vi "定点周期设置.vi"(4 "每月启动":T1, 6 "每周启动":T2, 7 "Display State In":T3, 8 "测量参数字符串[]":string[](array[string]), 9 "间隔启动":T9, 10 "定点周期":T6, 11 "周期模式":T5) -> (2 "保存输出":bool, 3 "周期设置输出":T8)   [LabVIEW 2016, in "定时设置.xctl"]
uses:
  <vilib>/Utility/miscctls.llb/LVPointTypeDef.ctl
panel:
  out "测试状态.结束时间":timestamp caption="结束时间" format="%<%y/%m/%d %H:%M:%S>T"
  out "测试状态.启动次数":dbl caption="启动次数"
  out "测试状态.启动时间":timestamp caption="启动时间" format="%<%y/%m/%d %H:%M:%S>T"
  in  "测量参数":T4 items=["氨氮"]
  in  "保存":bool
  in  "退出":bool
  in  "批量设置":bool
  out "周期模式选择卡":enum32{"选项卡 1", "选项卡 2"}(tab)
  # "分钟"
  # "次"
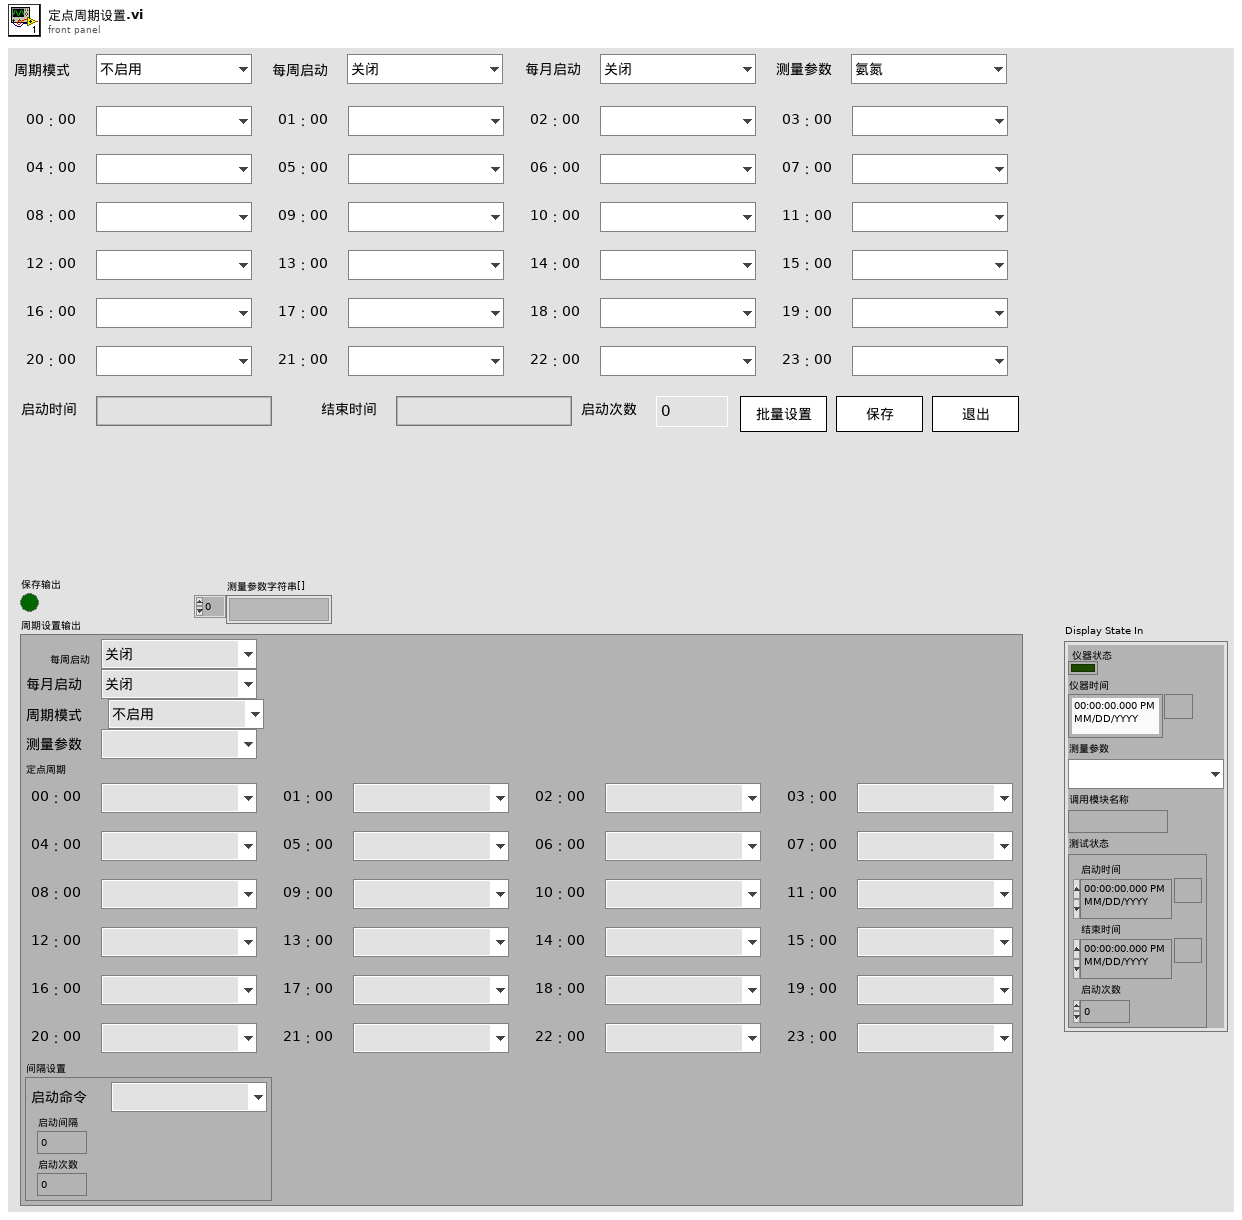
[diagram p1: front panel]
types:
  T1 = typedef "定时设置.xctl/每月启动.ctl" = enum16{"关闭", "1号", "2号", "3号", "4号", "5号", "6号", "7号", "8号", "9号", "10号", "11号", "12号", "13号", "14号", "15号", "16号", "17号", "18号", "19号", "20号", "21号", "22号", "23号", "24号", "25号", "26号", "27号", "28号", "29号", "30号", "31号"}
  T2 = typedef "定时设置.xctl/每周启动.ctl" = enum16{"关闭", "周日", "周一", "周二", "周三", "周四", "周五", "周六"}
  T3 = typedef "定时设置.xctl/状态 1.ctl" = cluster{"仪器状态":bool, "仪器时间":timestamp, "测量参数":T4, "调用模块名称":string, "测试状态":cluster{"启动时间":timestamp, "结束时间":timestamp, "启动次数":dbl}}
  T4 = typedef "定时设置.xctl/测量参数.ctl" = u16
  T5 = typedef "定时设置.xctl/周期模式设置.ctl" = enum16{"不启用", "定点模式", "间隔模式"}
  T6 = typedef "定时设置.xctl/定点周期设置.ctl" = cluster{"启动命令":T7, "启动命令 2":T7, "启动命令 3":T7, "启动命令 4":T7, "启动命令 5":T7, "启动命令 6":T7, "启动命令 7":T7, "启动命令 8":T7, "启动命令 9":T7, "启动命令 10":T7, "启动命令 11":T7, "启动命令 12":T7, "启动命令 13":T7, "启动命令 14":T7, "启动命令 15":T7, "启动命令 16":T7, "启动命令 17":T7, "启动命令 18":T7, "启动命令 19":T7, "启动命令 20":T7, "启动命令 21":T7, "启动命令 22":T7, "启动命令 23":T7, "启动命令 24":T7}
  T7 = typedef "定时设置.xctl/启动命令选择.ctl" = enum16{"", "水样测试", "标样核查", "零点核查", "跨度核查", "空白测试", "平行样测试", "加标回收", "空白校准", "标样校准", "初始化(清洗)"}
  T8 = cluster{"每周启动":T2, "每月启动":T1, "周期模式":T5, "测量参数":T4, "定点周期":T6, "间隔设置":cluster{"启动命令":T7, "启动间隔":dbl, "启动次数":i32}}
  T9 = typedef "定时设置.xctl/间隔启动设置.ctl" = cluster{"启动命令":T7, "启动间隔":dbl, "启动次数":i32}
  T10 = typedef "LVPointTypeDef.ctl" = cluster{"Horizontal":i16, "Vertical":i16}
  T11 = typedef "周期设置.lvlib/周期模式设置.ctl" = enum16{"不启用", "定点模式", "间隔模式"}
  T12 = cluster{"每周启动":T2, "每月启动":T1, "周期模式":T5, "测量参数":T4, "定点周期":T6, cluster{"启动命令":T7, "启动间隔":dbl, "启动次数":i32}}
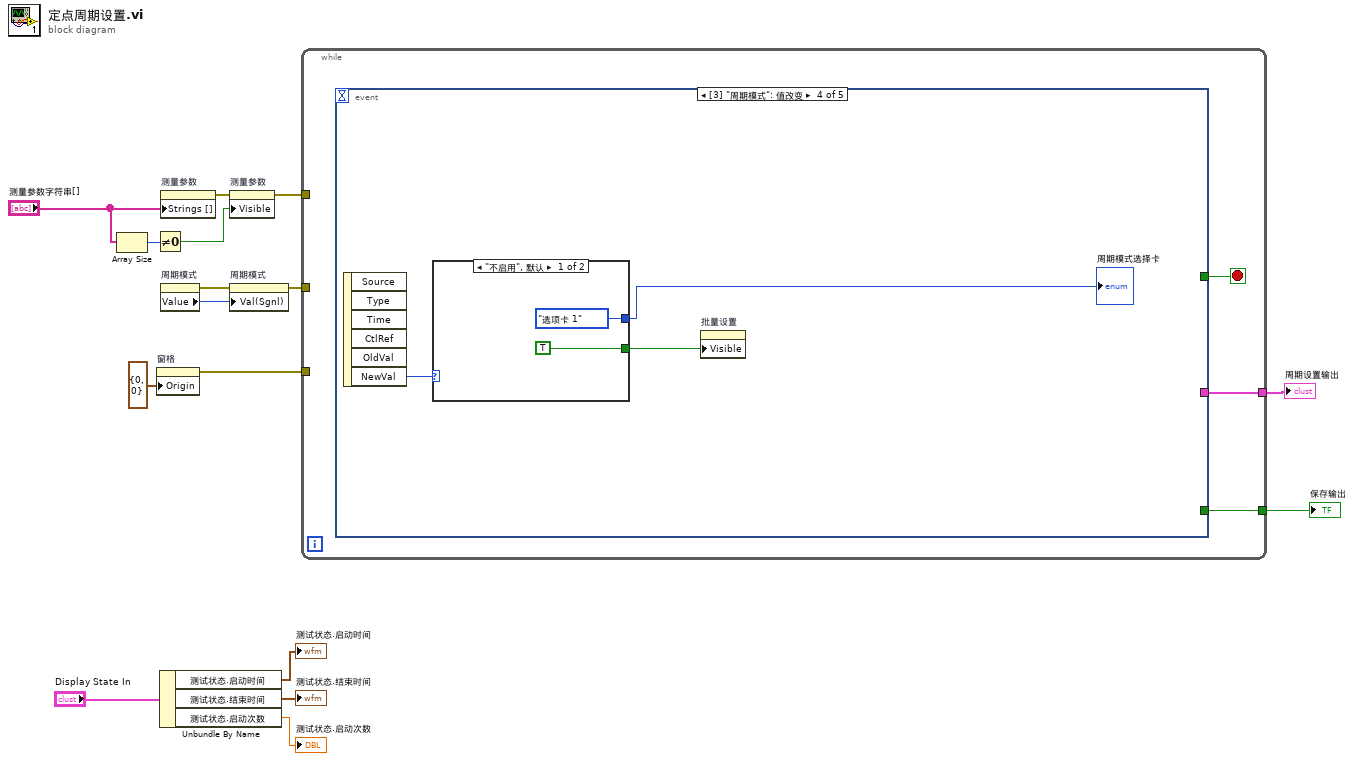
[diagram p0: block diagram]
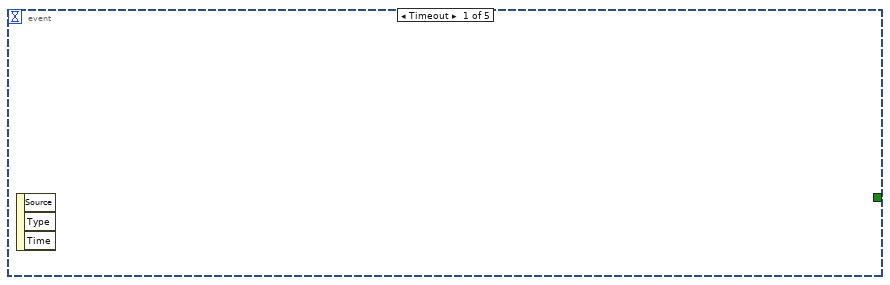
[diagram p2: hidden frame]
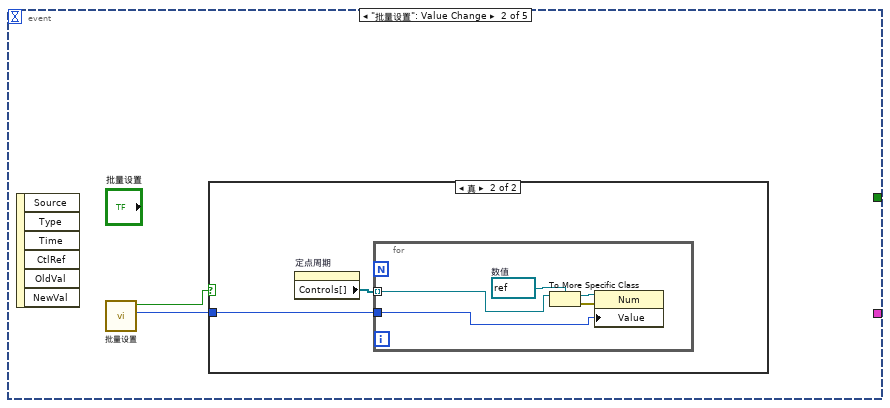
[diagram p3: hidden frame]
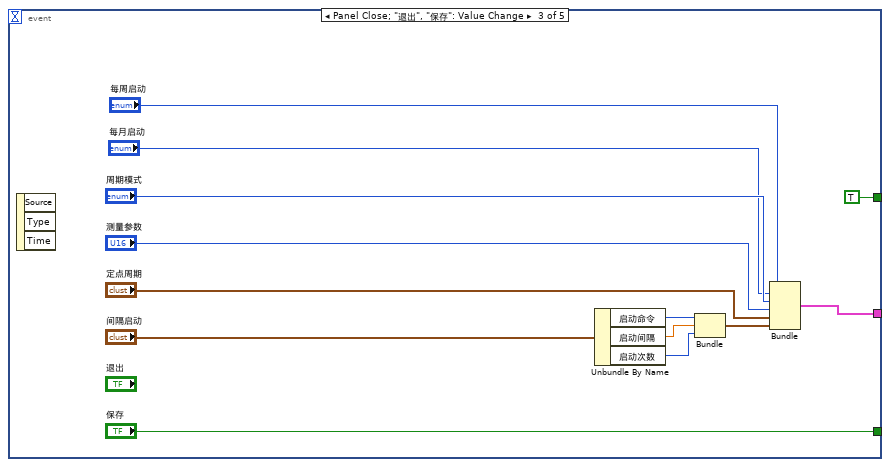
[diagram p5: hidden frame]
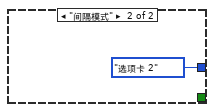
[diagram p6: hidden frame]
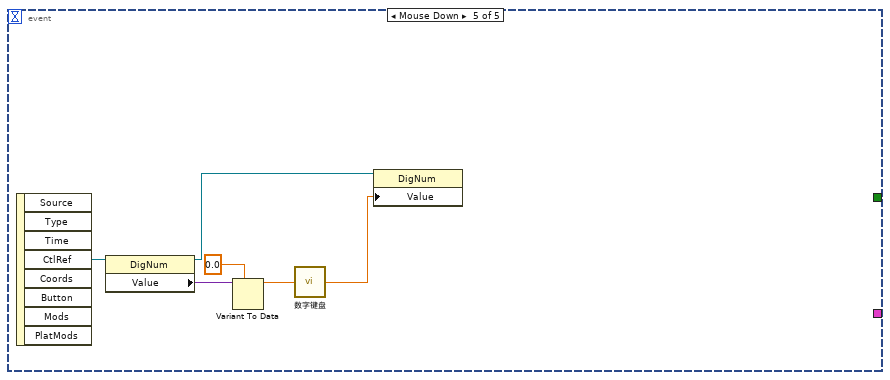
[diagram p7: hidden frame]
diagram:
  n1 = Array Size(array="测量参数字符串[]") -> (size(s)=w7:i32)
  n2 = Not Equal To 0?(x=w7) -> (x != 0?=w10:bool)
  n3 = property on="窗格" class="Pane"("Origin"=T10 {"Horizontal"=0, "Vertical"=0} ("原点")) -> (error out=w1:errorcluster)  [unwired: 2 in, 1 out]
  n4 = Unbundle By Name("Display State In") -> ("测试状态.启动时间"=→"测试状态.启动时间":timestamp, "测试状态.结束时间"=→"测试状态.结束时间":timestamp, "测试状态.启动次数"=→"测试状态.启动次数":dbl)
  n5 = property on="测量参数" class="Ring (严格)"("Strings []"="测量参数字符串[]") -> (error out=w11:errorcluster)  [unwired: 2 in, 1 out]
  n6 = property on="周期模式" class="Enum (严格)"() -> (error out=w15:errorcluster, "Value"=w16:T11)  [unwired: 2 in, 1 out]
  n7 = property on="测量参数" class="Ring (严格)"(error in=w11, "Visible"=w10) -> (error out=w9:errorcluster)  [unwired: 1 in, 1 out]
  n8 = property on="周期模式" class="Enum (严格)"(error in=w15, "Val(Sgnl)"=w16) -> (error out=w14:errorcluster)  [unwired: 1 in, 1 out]
  n9 = while {
    tunnel: [w18] -> w13
    tunnel: w14 -> [_]
    tunnel: [w17] -> w12
    tunnel: w9 -> [_]
    tunnel: w1 -> [_]
    stop <- w19 stop-if-true
    n10 = event shown="[3] \"周期模式\": 值改变" {
      selector: _ -> [_ _ _ _ _]
      dyn-events: _ -> [_ _ _ _ _]
      timeout: _ -> [_ _ _ _ _]
      tunnel: [_ _ TRUE _ _] -> w19
      tunnel: [_ _ w40 _ _] -> w18
      tunnel: [_ _ "保存" _ _] -> w17
      event Timeout {
        n11 = event-data() -> ()  [unwired: 1 in, 3 out]
      }
      event "批量设置": Value Change {
        n12 = event-data() -> ()  [unwired: 1 in, 6 out]
        n13 = call "批量设置.vi"() -> ("启动命令 2"=w21:T7, "确定 2"=w20:bool)  [unwired: 10 in]
        n14 = case shown="真" w20 {
          tunnel: w21 -> [_ w22]
          frame False {
          }
          frame True {
            n15 = property on="定点周期" class="Clust (严格)"() -> ("Controls[]"=w23:refnum<vi>[])  [unwired: 2 in, 2 out]
            n16 = for {
              tunnel: w23 -> [w28] mode=indexing
              tunnel: w22 -> [w24]
              w27 = refnum<vi> refnum  # 数值
              n17 = To More Specific Class(target class=w27, reference=w28) -> (specific class reference=w26:refnum<vi>, error out=w25:errorcluster)  [unwired: 1 in]
              n18 = property class="Num"(reference=w26, error in=w25, "Value"=w24) -> ()  [unwired: 2 out]
            }
          }
        }
      }
      event Panel Close; "退出", "保存": Value Change {
        n19 = event-data() -> ()  [unwired: 1 in, 3 out]
        n20 = Unbundle By Name("间隔启动") -> ("启动命令"=w37:T7, "启动间隔"=w36:dbl, "启动次数"=w35:i32)
        n21 = Bundle("启动命令"=w37, "启动间隔"=w36, "启动次数"=w35) -> (w34:cluster{"启动命令":T7, "启动间隔":dbl, "启动次数":i32})  [unwired: 1 in]
        n22 = Bundle("每周启动"="每周启动", "每月启动"="每月启动", "周期模式"="周期模式", "测量参数"="测量参数", "定点周期"="定点周期", w34) -> (w40:T12)  [unwired: 1 in]
      }
      event Value Change {
        n23 = event-data() -> ("NewVal"=w43:T5)  [unwired: 1 in, 5 out]
        n24 = case shown="\"不启用\", 默认" w43 {
          tunnel: [TRUE ("可见") _] -> w44
          tunnel: [enum32{"选项卡 1", "选项卡 2"}."选项卡 1" ("周期模式选择卡") enum32{"选项卡 1", "选项卡 2"}."选项卡 2" ("周期模式选择卡")] -> w42
          frame "不启用", Default {
          }
          frame "间隔模式" {
          }
        }
        "周期模式选择卡" <- w42
        n25 = property on="批量设置" class="Bool"("Visible"=w44) -> ()  [unwired: 2 in, 2 out]
      }
      event Mouse Down {
        n26 = event-data() -> ("CtlRef"=w53:refnum<vi>)  [unwired: 1 in, 7 out]
        n27 = property class="DigNum"(reference=w53) -> (reference out=w52:refnum<vi>, "Value"=w51:variant)  [unwired: 1 in, 1 out]
        n28 = Variant To Data(type=0.0, Variant=w51) -> (data=w49:dbl)  [unwired: 1 in, 1 out]
        n29 = call "数字键盘.vi"("OldNumber"=w49) -> ("NewNumber"=w48:sgl)
        n30 = property class="DigNum"(reference=w52, "Value"=w48) -> ()  [unwired: 1 in, 2 out]
      }
    }
  }
  "周期设置输出" <- w13
  "保存输出" <- w12
